vi "Day 12-1.vi"() -> ()   [LabVIEW 2019, in "Day 12.lvlib"]
uses:
  Day 12.lvlib
  Controls/Cave.ctl
  Controls/Cave Type.ctl
panel:
  out "Posible routes":i32[](array[numeric])
  out "Valid routes":T1[][](array[typedef])
  out "Caves":T1[](array[typedef])
  in  "String":string
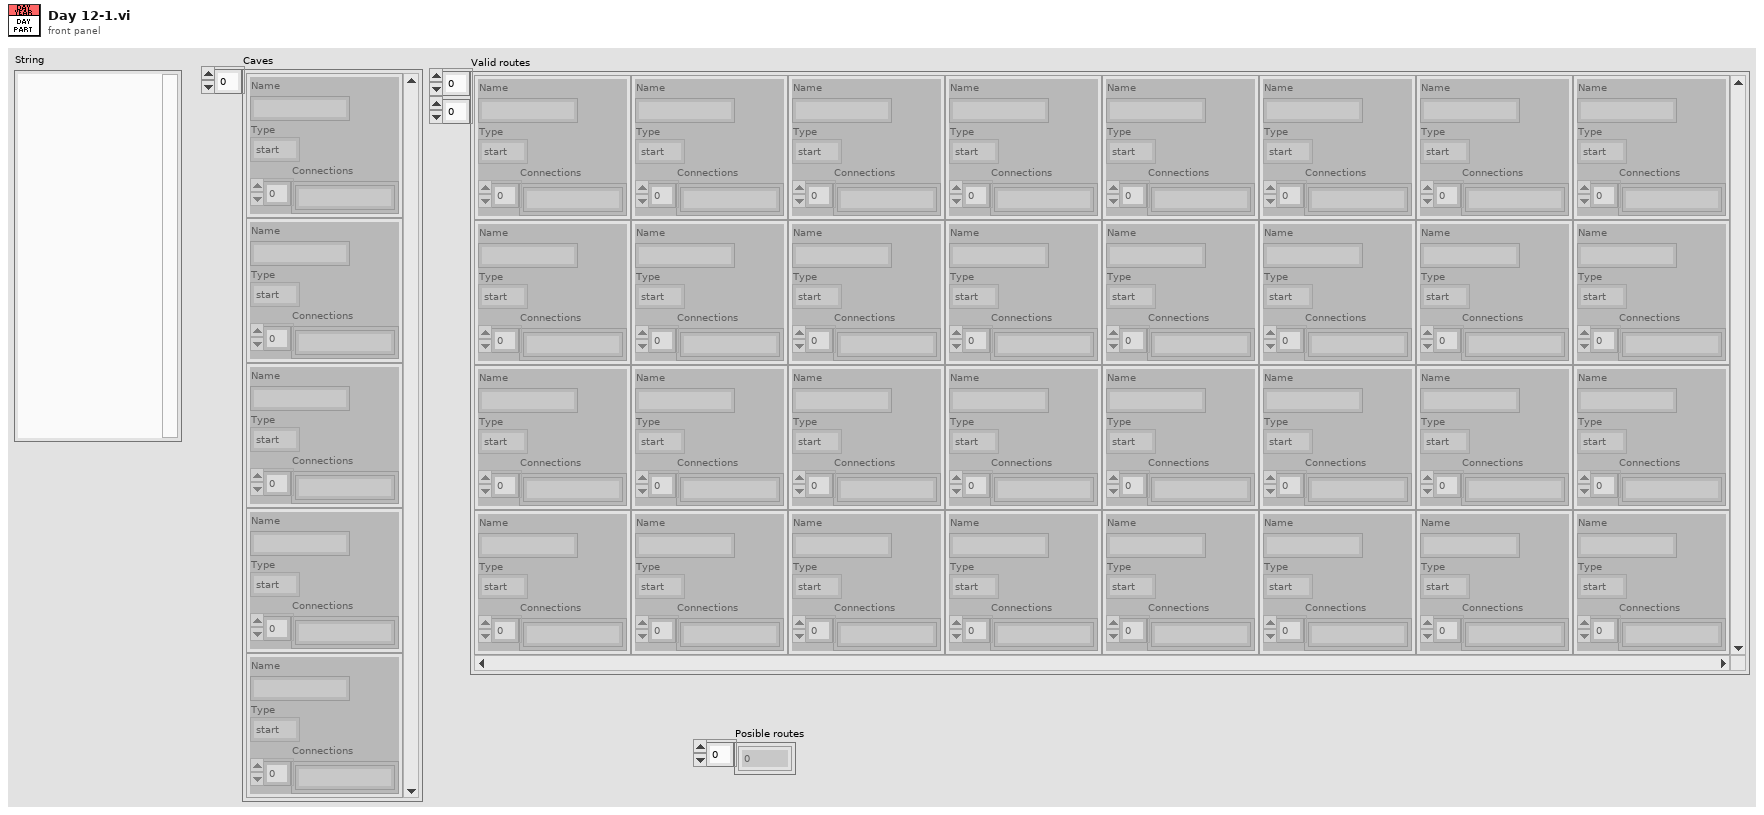
[diagram p1: front panel]
types:
  T1 = typedef "Day 12.lvlib/Cave.ctl" = cluster{"Name":string, "Type":T2, "Connections":string[]}
  T2 = typedef "Day 12.lvlib/Cave Type.ctl" = enum16{"start", "end", "small", "big"}
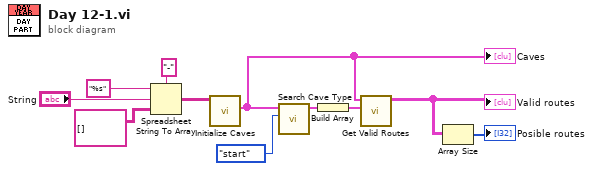
[diagram p0: block diagram]
diagram:
  n1 = Spreadsheet String To Array(delimiter (Tab)="-", format string="%s", spreadsheet string="String", array type (2D Dbl)=string[][] []) -> (array=w7:string[][])
  n2 = call "Initialize Caves.vi"("array type (2D Dbl)"=w7) -> ("Array"=w4:T1[])  [unwired: 9 in, 1 out]
  "Caves" <- w4
  n3 = call "Search Cave Type.vi"("Type"=Cave_Type."start", "Array"=w4) -> ("Cave"=w5:T1)  [unwired: 8 in, 1 out]
  n4 = Build Array(w5) -> (w3:T1[])
  n5 = call "Get Valid Routes.vi"("Starting Route"=w3, "All Caves"=w4) -> ("Ended Valid Routes Out"=w2:T1[][])  [unwired: 9 in]
  "Valid routes" <- w2
  n6 = Array Size(array=w2) -> (size(s)=→"Posible routes":i32[])
